vi "Read Data.vi"(5 "CS (None)":refnum<class "SPI CS.lvclass">, 7 "SPI":refnum<class "SPI.lvclass">, 8 "error in (no error)":errorcluster, 9 "Len":u8, 11 "Session In":refnum<class "Session.lvclass">) -> (0 "error out":errorcluster, 1 "Data":string, 3 "Session Out":refnum<class "Session.lvclass">)   [LabVIEW 2020, in "CTI.lvlib" / "SPI.lvclass"]
uses:
  SPI.lvclass/SPI.ctl
  SPI.lvclass
  Session/Session.lvclass
  SPI CS/SPI CS.lvclass
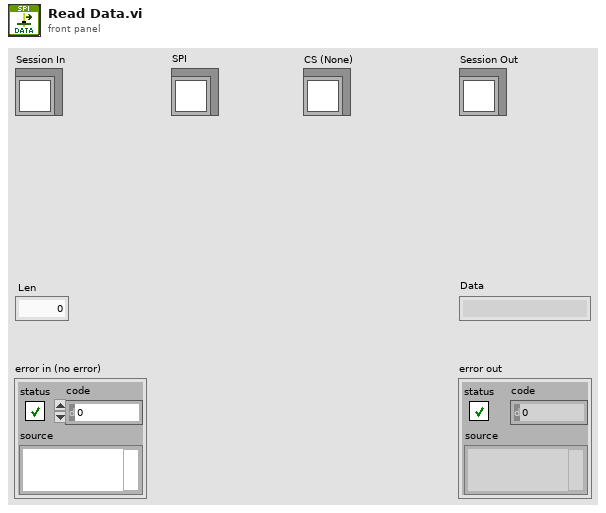
[diagram p1: front panel]
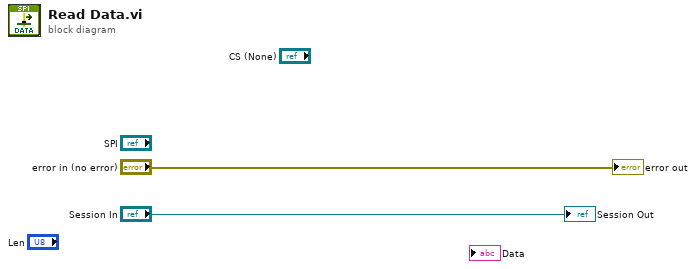
[diagram p0: block diagram]
diagram:
  "error out" <- "error in (no error)"
  "Session Out" <- "Session In"
